vi "SeCrTs-Login_Main.vi"(8 "error in":errorcluster) -> (0 "error out":errorcluster, 3 "Login pass":bool)   [LabVIEW 2022 SP3]
uses:
  <vilib>/Utility/error.llb/Trim Whitespace One-Sided.vi
  <vilib>/Utility/file.llb/Read Delimited Spreadsheet (string).vi
  <vilib>/Utility/file.llb/Write Delimited Spreadsheet (string).vi
panel:
  in  "Log In Tool":bool
  in  "Enter":bool
  in  "Stop Button":bool
  out "Pass = True":bool
  in  "Change Password":bool
  in  "Show Password":bool
  in  "Password":string
  in  "Select User":u16(ring) items=["Vigneshwaran", "Kannan", "Arul"]
  # "Agnikul Cosmos"
  # "User Login"
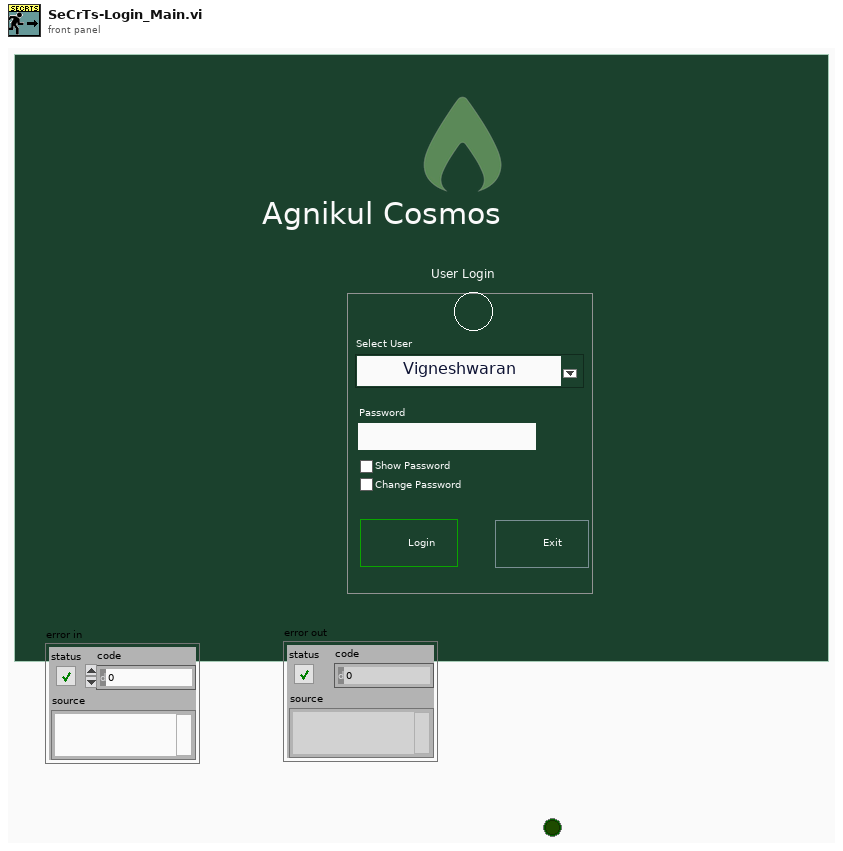
[diagram p1: front panel]
types:
  T1 = typedef "SeCrTs-file folder ctl.ctl" = cluster{"Datalog path":path, "Configuration path":path, "Signal list path":path, "Sub vi's":path, "Authentication":path, "Sequence":path, "Event Log":path, "CS Error log":path, "RT Error Log":path}
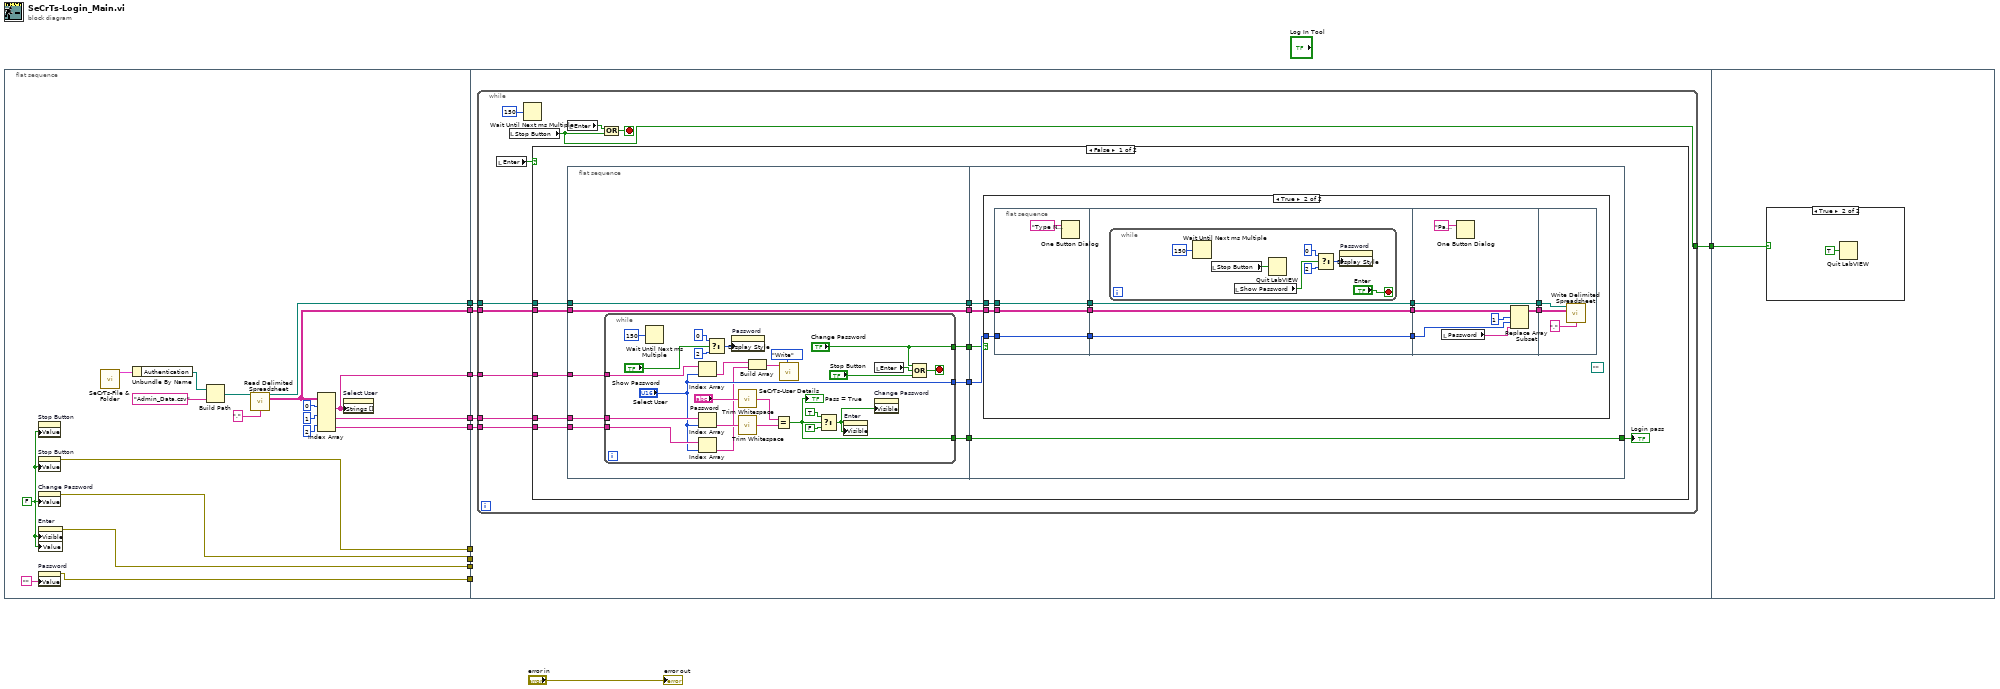
[diagram p0: block diagram]
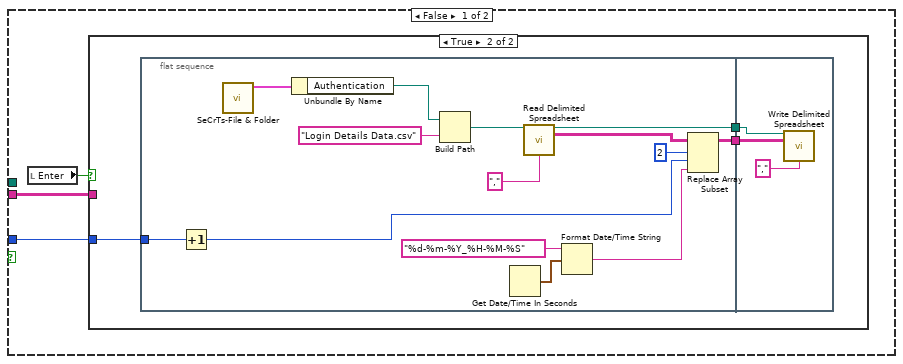
[diagram p2: hidden frame]
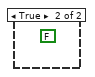
[diagram p4: hidden frame]
diagram:
  n1 = flat-sequence {
    tunnel: [w28] -> w11
    tunnel: [w24] -> w10
    tunnel: [w20] -> w9
    tunnel: [w27] -> w8
    tunnel: [w25] -> w7
    tunnel: [w22] -> w6
    tunnel: [w21] -> w5
    tunnel: [w19] -> w4
    tunnel: [w14] -> w3
    tunnel: w5 -> [_]
    tunnel: w6 -> [_]
    tunnel: w7 -> [w34]
    tunnel: w8 -> [_]
    tunnel: w9 -> [_]
    tunnel: w10 -> [w35]
    tunnel: w11 -> [w36]
    tunnel: w4 -> [w33]
    tunnel: w3 -> [w32]
    tunnel: [w31] -> w2
    tunnel: w2 -> [w154]
    frame #0 {
      w12 = FALSE ("Change Password")
      n2 = property on="Stop Button" class="Bool (strict)"("Value"=w12) -> ()  [unwired: 2 in, 2 out]
      n3 = property on="Stop Button" class="Bool (strict)"("Value"=w12) -> (error out=w21:errorcluster)  [unwired: 2 in, 1 out]
      n4 = property on="Change Password" class="Bool (strict)"("Value"=w12) -> (error out=w27:errorcluster)  [unwired: 2 in, 1 out]
      n5 = property on="Enter" class="Bool (strict)"("Visible"=w12, "Value"=w12) -> (error out=w20:errorcluster)  [unwired: 2 in, 1 out]
      n6 = property on="Password" class="Str"("Value"="") -> (error out=w22:errorcluster)  [unwired: 2 in, 1 out]
      n7 = call "SeCrTs-File & Folder.vi"() -> ("File Output"=w17:T1)  [unwired: 10 in, 1 out]
      n8 = Unbundle By Name(w17) -> ("Authentication"=w16:path)
      n9 = Build Path(base path=w16, name or relative path="Admin_Data.csv" ("name")) -> (appended path=w18:path)
      n10 = call-poly <vilib>:"Read Delimited Spreadsheet.vi"("file path (dialog if empty)"=w18, "delimiter (\\t)"="," ("delimiter (\\t)")) -> ("new file path (Not A Path if cancelled)"=w25:path, "all rows"=w24:string[][])  [unwired: 8 in, 4 out]
      n11 = Index Array(array=w24, index (row) #1=0 ("index (row)"), index (row) #2=1 ("index (row)"), index (row) #3=2 ("disabled index (col)")) -> (element #1=w19:string[], element #2=w28:string[], element #3=w14:string[])  [unwired: 3 in]
      n12 = property on="Select User" class="Ring (strict)"("Strings []"=w19) -> ()  [unwired: 2 in, 2 out]
    }
    frame #1 {
      n13 = while {
        tunnel: w36 -> [w45]
        tunnel: w35 -> [w44]
        tunnel: w34 -> [w43]
        tunnel: w33 -> [w41]
        tunnel: w32 -> [w40]
        tunnel: [w37] -> w31
        stop <- w39 stop-if-true
        n14 = local read "Enter"() -> (w42:bool)
        n15 = local read "Stop Button"() -> (w37:bool)
        n16 = Wait Until Next ms Multiple(millisecond multiple=u32 150) -> ()  [unwired: 1 out]
        n17 = case shown="False" w42 {
          tunnel: w45 -> [w55 _]
          tunnel: w44 -> [w54 _]
          tunnel: w43 -> [w51 _]
          tunnel: w41 -> [w50 _]
          tunnel: w40 -> [w49 _]
          frame False {
            n18 = flat-sequence {
              tunnel: [w65] -> w57
              tunnel: [w64] -> w56
              tunnel: w54 -> [w65]
              tunnel: w55 -> [w63]
              tunnel: [w62] -> w53
              tunnel: [w61] -> w52
              tunnel: w51 -> [w61]
              tunnel: w50 -> [w60]
              tunnel: w49 -> [w59]
              tunnel: [w58] -> w48
              tunnel: w57 -> [w95]
              tunnel: w56 -> [w94]
              tunnel: w53 -> [w93]
              tunnel: w52 -> [w92]
              tunnel: w48 -> [w91]
              tunnel: [w91] -> w47
              frame #0 {
                n19 = while {
                  tunnel: ["Select User"] -> w64
                  tunnel: w63 -> [w90]
                  tunnel: ["Change Password"] -> w62
                  tunnel: w60 -> [w74]
                  tunnel: w59 -> [w73]
                  tunnel: [w70] -> w58
                  stop <- w79 stop-if-true
                  n20 = Wait Until Next ms Multiple(millisecond multiple=u32 150) -> ()  [unwired: 1 out]
                  n21 = Index Array(array=w74, index="Select User") -> (element=w68:string)
                  n22 = Index Array(array=w90, index="Select User") -> (element=w89:string)
                  n23 = Index Array(array=w73, index="Select User") -> (element=w67:string)
                  n24 = Select(t=u32 0 ("Display Style"), s="Show Password", f=u32 2 ("Display Style")) -> (s? t:f=w83:u32)
                  n25 = property on="Password" class="Str"("Display Style"=w83) -> ()  [unwired: 2 in, 2 out]
                  n26 = call <vilib>:"Trim Whitespace.vi"("string"="Password") -> ("trimmed string"=w85:string)  [unwired: 1 in]
                  n27 = call <vilib>:"Trim Whitespace.vi"("string"=w89) -> ("trimmed string"=w75:string)  [unwired: 1 in]
                  n28 = Build Array(w68, w67) -> (w66:string[])
                  n29 = Equal?(x=w85, y=w75) -> (x = y?=w70:bool)
                  "Pass = True" <- w70
                  n30 = call "SeCrTs-User Details.vi"("Enum"=enum16{"Read", "Write"}."Write", "User details"=w66) -> ()  [unwired: 8 in, 2 out]
                  n31 = Select(t=TRUE, s=w70, f=FALSE ("Visible")) -> (s? t:f=w76:bool)
                  n32 = property on="Enter" class="Bool (strict)"("Visible"=w76) -> ()  [unwired: 2 in, 2 out]
                  n33 = local read "Enter"() -> (w77:bool)
                  n34 = property on="Change Password" class="Bool (strict)"("Visible"=w76) -> ()  [unwired: 2 in, 2 out]
                  n35 = Compound Arithmetic op=OR("Change Password", w77, "Stop Button") -> (w79:bool)
                }
              }
              frame #1 {
                n36 = case shown="True" w93 {
                  tunnel: w95 -> [w98 w127]
                  tunnel: w94 -> [w97 w124]
                  tunnel: w92 -> [_ w119]
                  frame False {
                    n37 = local read "Enter"() -> (w96:bool)
                    n38 = case shown="True" w96 {
                      tunnel: w98 -> [_ _]
                      tunnel: w97 -> [_ w101]
                      frame False {
                      }
                      frame True {
                        n39 = flat-sequence {
                          tunnel: w101 -> [w115]
                          tunnel: [w105] -> w100
                          tunnel: [w104] -> w99
                          tunnel: w100 -> [w117]
                          tunnel: w99 -> [w118]
                          frame #0 {
                            n40 = Increment(x=w115) -> (x+1=w108:u16)
                            n41 = call "SeCrTs-File & Folder.vi"() -> ("File Output"=w111:T1)  [unwired: 10 in, 1 out]
                            n42 = Unbundle By Name(w111) -> ("Authentication"=w110:path)
                            n43 = Build Path(base path=w110, name or relative path="Login Details Data.csv" ("name")) -> (appended path=w107:path)
                            n44 = Get Date/Time In Seconds() -> (seconds since 1Jan1904=w102:timestamp)
                            n45 = call-poly <vilib>:"Read Delimited Spreadsheet.vi"("file path (dialog if empty)"=w107, "delimiter (\\t)"="," ("delimiter (\\t)")) -> ("new file path (Not A Path if cancelled)"=w104:path, "all rows"=w106:string[][])  [unwired: 8 in, 4 out]
                            n46 = Format Date/Time String(time format string (%c)="%d-%m-%Y_%H-%M-%S", seconds (now)=w102) -> (date/time string=w113:string)  [unwired: 1 in]
                            n47 = Replace Array Subset(array=w106, new element=w113, index (row)=2, index (col)=w108) -> (w105:string[][])
                          }
                          frame #1 {
                            n48 = call-poly <vilib>:"Write Delimited Spreadsheet.vi"("file path (dialog if empty)"=w118, "2D data"=w117, "delimiter (\\t)"="," ("delimiter (\\t)")) -> ()  [unwired: 11 in, 2 out]
                          }
                        }
                      }
                    }
                  }
                  frame True {
                    (unwired) path "" ("new file path (Not A Path if cancelled)")
                    n49 = flat-sequence {
                      tunnel: [w133] -> w128
                      tunnel: w127 -> [w133]
                      tunnel: [w132] -> w125
                      tunnel: w124 -> [w132]
                      tunnel: [w131] -> w120
                      tunnel: w119 -> [w131]
                      tunnel: [w136] -> w129
                      tunnel: w128 -> [w136]
                      tunnel: [w135] -> w126
                      tunnel: w125 -> [w135]
                      tunnel: [w134] -> w121
                      tunnel: w120 -> [w134]
                      tunnel: w129 -> [w149]
                      tunnel: w126 -> [w147]
                      tunnel: [w145] -> w123
                      tunnel: [w144] -> w122
                      tunnel: w121 -> [w144]
                      tunnel: w123 -> [w153]
                      tunnel: w122 -> [w152]
                      frame #0 {
                        n50 = One Button Dialog(message="Type New Password and Press Enter button") -> ()  [unwired: 1 in, 1 out]
                      }
                      frame #1 {
                        n51 = while {
                          stop <- "Enter" stop-if-true
                          n52 = Wait Until Next ms Multiple(millisecond multiple=u32 150) -> ()  [unwired: 1 out]
                          n53 = local read "Stop Button"() -> (w142:bool)
                          n54 = local read "Show Password"() -> (w137:bool)
                          n55 = Quit LabVIEW(quit? (T)=w142) -> ()
                          n56 = Select(t=u32 0 ("Display Style"), s=w137, f=u32 2 ("Display Style")) -> (s? t:f=w138:u32)
                          n57 = property on="Password" class="Str"("Display Style"=w138) -> ()  [unwired: 2 in, 2 out]
                        }
                      }
                      frame #2 {
                        n58 = local read "Password"() -> (w146:string)
                        n59 = One Button Dialog(message="Password changed successfully, Please Login with new Password") -> ()  [unwired: 1 in, 1 out]
                        n60 = Replace Array Subset(array=w149, new element=w146, index (row)=1, index (col)=w147) -> (w145:string[][])
                      }
                      frame #3 {
                        n61 = call-poly <vilib>:"Write Delimited Spreadsheet.vi"("file path (dialog if empty)"=w152, "2D data"=w153, "delimiter (\\t)"="," ("delimiter (\\t)")) -> ()  [unwired: 11 in, 2 out]
                      }
                    }
                  }
                }
              }
            }
            "Login pass" <- w47
          }
          frame True {
            (unwired) FALSE
          }
        }
        n62 = local read "Enter"() -> (w38:bool)
        n63 = Compound Arithmetic op=OR(w38, w37) -> (w39:bool)
      }
    }
    frame #2 {
      n64 = case shown="True" w154 {
        frame False {
        }
        frame True {
          n65 = Quit LabVIEW(quit? (T)=TRUE) -> ()
        }
      }
    }
  }
  "error out" <- "error in"
